vi "RT_pid_autotune.vi"() -> ()   [LabVIEW 2018]
uses:
  <vilib>/addons/control/pid/autopid.llb/PID autotuning parameters (adv).ctl
  <vilib>/FPGAPlugInAG/myRIO-1900/niLvFpga_Open_myRIO-1900.vi
  <vilib>/rvi/interface/common/dynamic/niFpgaDynamicAddResources.vi
  <vilib>/Utility/error.llb/Error Cluster From Error Code.vi
  <vilib>/rvi/errors/niLvFpgaAdjustHostInterfaceError.vi
  <vilib>/FPGAPlugInAG/Dynamic/niLvFpga_Close_Dynamic.vi
  <vilib>/rvi/interface/nirviOpenFPGA/nirviOpenFPGA.xnode
  FPGA Bitfiles/DQNcarpolelvsim_FPGATarget_FPGAsmall2_-ePuv6MPJ4E.lvbitx
  FPGA_small2.vi
  <vilib>/rvi/interface/nirviReadWriteControl/nirviReadWriteControl.xnode
  <vilib>/rvi/interface/nirviCloseFPGA/nirviCloseFPGA.xnode
  NiFpgaLv.dll
  <vilib>/rvi/interface/Simulation/niFpgaSimulationCallBeginRW.vi
  <vilib>/addons/control/pid/NI_PID_autopid.lvlib
panel:
  in  "auto? (F)":bool
  in  "autotuning parameters":T1={"technique"=2, "type of controller"=1, "control specification"=0, "amplitude"=1.0} {"amplitude" format="%.2f"; "control specification" items=["normal", "fast", "slow"]; "type of controller" items=["P", "PI", "PID"]; "technique" items=["Step Open Loop", "Step Closed Loop", "Relay", "PID Relay"]}
  in  "autotune? (F)":bool
  in  "set_point":i16(slide)=207 scale=-800.0..800.0
  in  "stop":bool
  out "position":i16=209
  out "speed Chart":i16(graph)
  in  "PID gains":T2={"proportional gain (Kc)"=0.0005, "integral time (Ti, min)"=0.001, "derivative time (Td, min)"=0.001} {"derivative time (Td, min)" format="%.5f"; "integral time (Ti, min)" format="%.4f"; "proportional gain (Kc)" format="%.4f"}
  in  "dt (s)":dbl=0.001 format="%.3f"
  in  "output range":cluster{"output high":dbl, "output low":dbl}={"output high"=700.0, "output low"=550.0} {"output low" format="%.2f"; "output high" format="%.2f"}
  out "output":dbl=559.250913333665 format="%.2f"
  out "off_track":bool
  out "busy":bool
  out "states":dbl[](array[numeric])
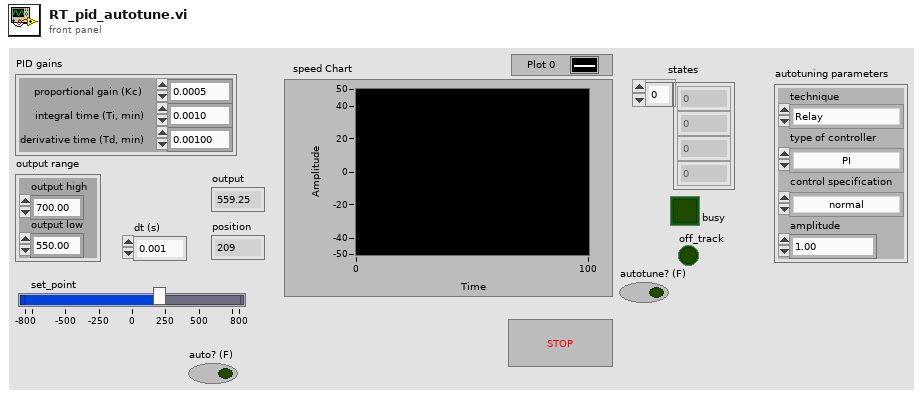
[diagram p1: front panel]
types:
  T1 = typedef "NI_PID_autopid.lvlib/PID autotuning parameters (adv).ctl" = cluster{"technique":u16, "type of controller":u16, "control specification":u16, "amplitude":dbl}
  T2 = cluster{"proportional gain (Kc)":dbl, "integral time (Ti, min)":dbl, "derivative time (Td, min)":dbl}
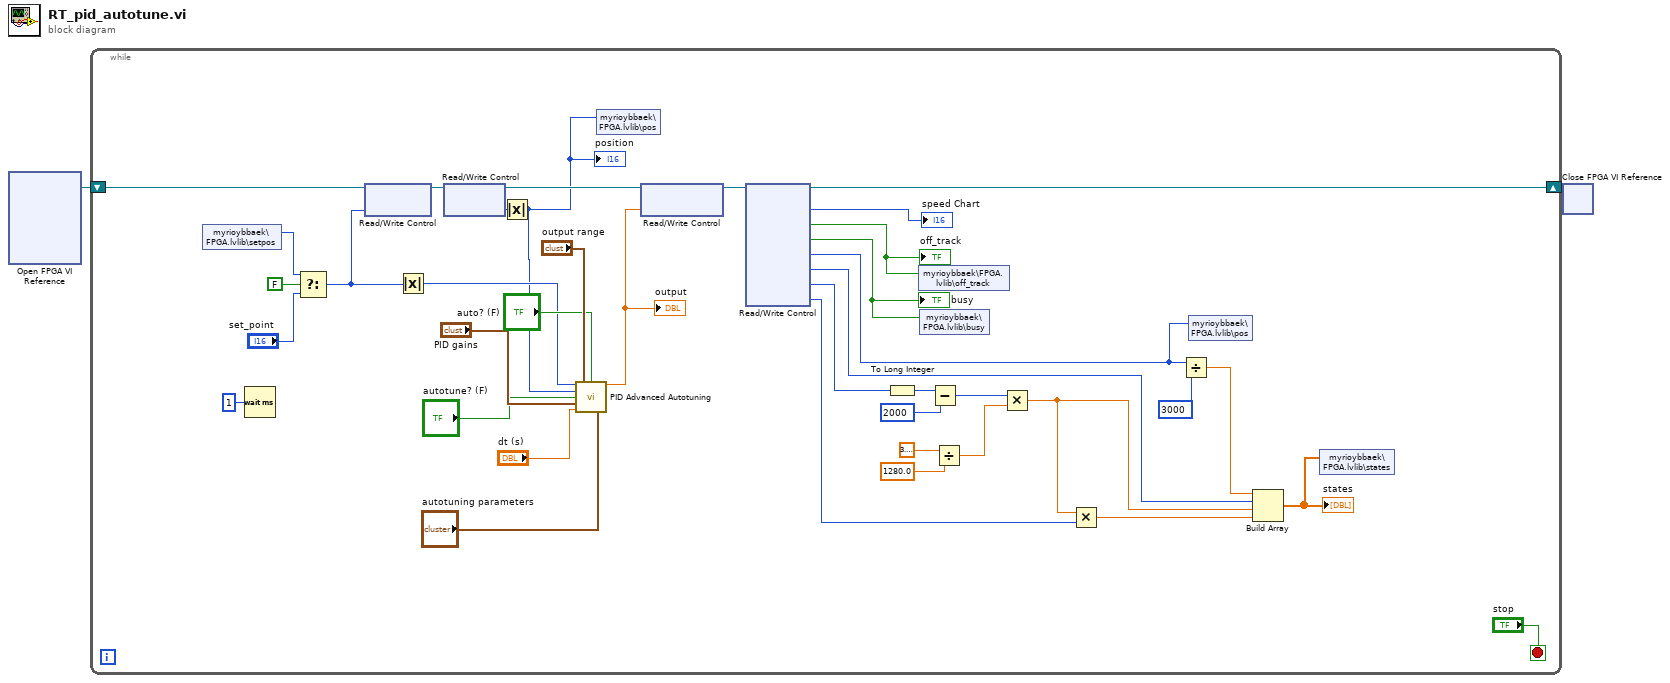
[diagram p0: block diagram]
diagram:
  n1 = xnode "Open FPGA VI Reference"() -> ("FPGA VI Reference Out"=w2:refnum<k20>)  [unwired: 2 in, 1 out]
  n2 = while {
    shift-right: [w34] -> w1
    shift-left: w2 -> [w41]
    stop <- "stop" stop-if-true
    n3 = shared-variable "myrioybbaek\\FPGA.lvlib\\setpos"() -> (w32:i16)  [unwired: 1 in, 1 out]
    n4 = Wait (ms)(milliseconds to wait=u32 1) -> ()  [unwired: 1 out]
    n5 = Select(t=w32, s=FALSE, f="set_point") -> (s? t:f=w11:i16)
    n6 = xnode "Read/Write Control"("FPGA VI Reference In"=w41, "set_point"=w11) -> ("FPGA VI Reference Out"=w38:refnum<k20>)  [unwired: 1 in, 1 out]
    n7 = Absolute Value(x=w11) -> (abs(x)=w4:i16)
    n8 = xnode "Read/Write Control"("FPGA VI Reference In"=w38) -> ("FPGA VI Reference Out"=w37:refnum<k20>, "position"=w10:i16)  [unwired: 1 in, 1 out]
    n9 = Absolute Value(x=w10) -> (abs(x)=w3:i16)
    "position" <- w3
    n10 = call <vilib>:"PID Advanced Autotuning.vi"("setpoint"=w4, "output range"="output range", "auto? (F)"="auto? (F)", "process variable"=w3, "autotune? (F)"="autotune? (F)", "PID gains"="PID gains", "dt (s)"="dt (s)", "autotuning parameters"="autotuning parameters") -> ("output"=w8:dbl)  [unwired: 5 in, 2 out]
    "output" <- w8
    n11 = shared-variable "myrioybbaek\\FPGA.lvlib\\pos"(w3) -> ()  [unwired: 1 in, 1 out]
    n12 = xnode "Read/Write Control"("FPGA VI Reference In"=w37, "dt_pwm_ms"=w8) -> ("FPGA VI Reference Out"=w36:refnum<k20>)  [unwired: 1 in, 1 out]
    n13 = xnode "Read/Write Control"("FPGA VI Reference In"=w36) -> ("FPGA VI Reference Out"=w34:refnum<k20>, "speed"=→"speed Chart":i16, "off_track"=w30:bool, "busy"=w17:bool, "position"=w18:i16, "speed"=w15:i16, "AI0"=w16:u16, "dAI"=w14:i16)  [unwired: 1 in, 1 out]
    "off_track" <- w30
    "busy" <- w17
    n14 = To Long Integer(number=w16) -> (32bit integer=w29:i32)
    n15 = shared-variable "myrioybbaek\\FPGA.lvlib\\off_track"(w30) -> ()  [unwired: 1 in, 1 out]
    n16 = shared-variable "myrioybbaek\\FPGA.lvlib\\busy"(w17) -> ()  [unwired: 1 in, 1 out]
    n17 = Subtract(x=w29, y=u16 2000) -> (x-y=w27:i32)
    n18 = Divide(x=3.141592653589793, y=1280.0) -> (x/y=w28:dbl)
    n19 = Multiply(x=w27, y=w28) -> (x*y=w25:dbl)
    n20 = Multiply(x=w25, y=w14) -> (x*y=w26:dbl)
    n21 = Divide(x=w18, y=i16 3000) -> (x/y=w21:dbl)
    n22 = shared-variable "myrioybbaek\\FPGA.lvlib\\pos"(w18) -> ()  [unwired: 1 in, 1 out]
    n23 = Build Array(w21, w15, w25, w26) -> (w19:dbl[])
    "states" <- w19
    n24 = shared-variable "myrioybbaek\\FPGA.lvlib\\states"(w19) -> ()  [unwired: 1 in, 1 out]
  }
  n25 = xnode "Close FPGA VI Reference"("FPGA VI Reference In"=w1) -> ()  [unwired: 1 in, 1 out]
